vi "DCMotor_WithReduction.vi"(9 "GearBoxReduction":dbl=1.0 format="%13.5p", 11 "in DCMOTOR":T1 {"Jr_KgM2" format="%13.5p"; "L_H" format="%13.5p"; "Kt_NMPerAmp" format="%13.5p"; "KvINV_RadPerSecPerVolt" format="%13.5p"; "R_Ohms" format="%13.5p"; "FreeSpeed_RadPerSec" format="%13.5p"; "FreeCurrent_Amps" format="%13.5p"; "StallCurrent_Amps" format="%13.5p"; "StallTorque_NM" format="%13.5p"; "nominalVoltage_Volts" format="%13.5p"}) -> (3 "out DCMOTOR":T1 {"Jr_KgM2" format="%13.5p"; "L_H" format="%13.5p"; "Kt_NMPerAmp" format="%13.5p"; "KvINV_RadPerSecPerVolt" format="%13.5p"; "R_Ohms" format="%13.5p"; "FreeSpeed_RadPerSec" format="%13.5p"; "FreeCurrent_Amps" format="%13.5p"; "StallCurrent_Amps" format="%13.5p"; "StallTorque_NM" format="%13.5p"; "nominalVoltage_Volts" format="%13.5p"})   [LabVIEW 2019, in "Trajectory_Library.lvlib"]
doc: "Returns a copy of this motor with the given gearbox reduction applied.\n\nInputs: \n - in DCMOTOR -- Cluster containing the motor modeling constants for this set of motors.\n - GearboxReduction -- double -- The gearbox reduction.\n\nOutputs:\n - out DCMOTOR -- Revised cluster containing the motor modeling constants for this set of motors."
uses:
  Trajectory_Library.lvlib
  TypeDef/DCMOTOR.CTL
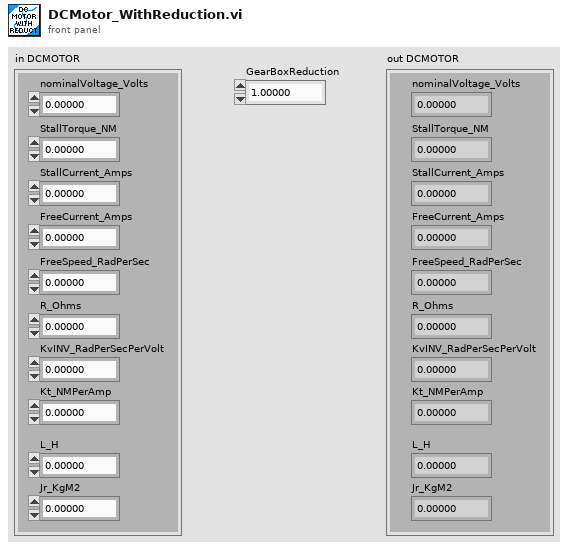
[diagram p1: front panel]
types:
  T1 = typedef "Trajectory_Library.lvlib/DCMOTOR.CTL" = cluster{"nominalVoltage_Volts":dbl, "StallTorque_NM":dbl, "StallCurrent_Amps":dbl, "FreeCurrent_Amps":dbl, "FreeSpeed_RadPerSec":dbl, "R_Ohms":dbl, "KvINV_RadPerSecPerVolt":dbl, "Kt_NMPerAmp":dbl, "L_H":dbl, "Jr_KgM2":dbl}
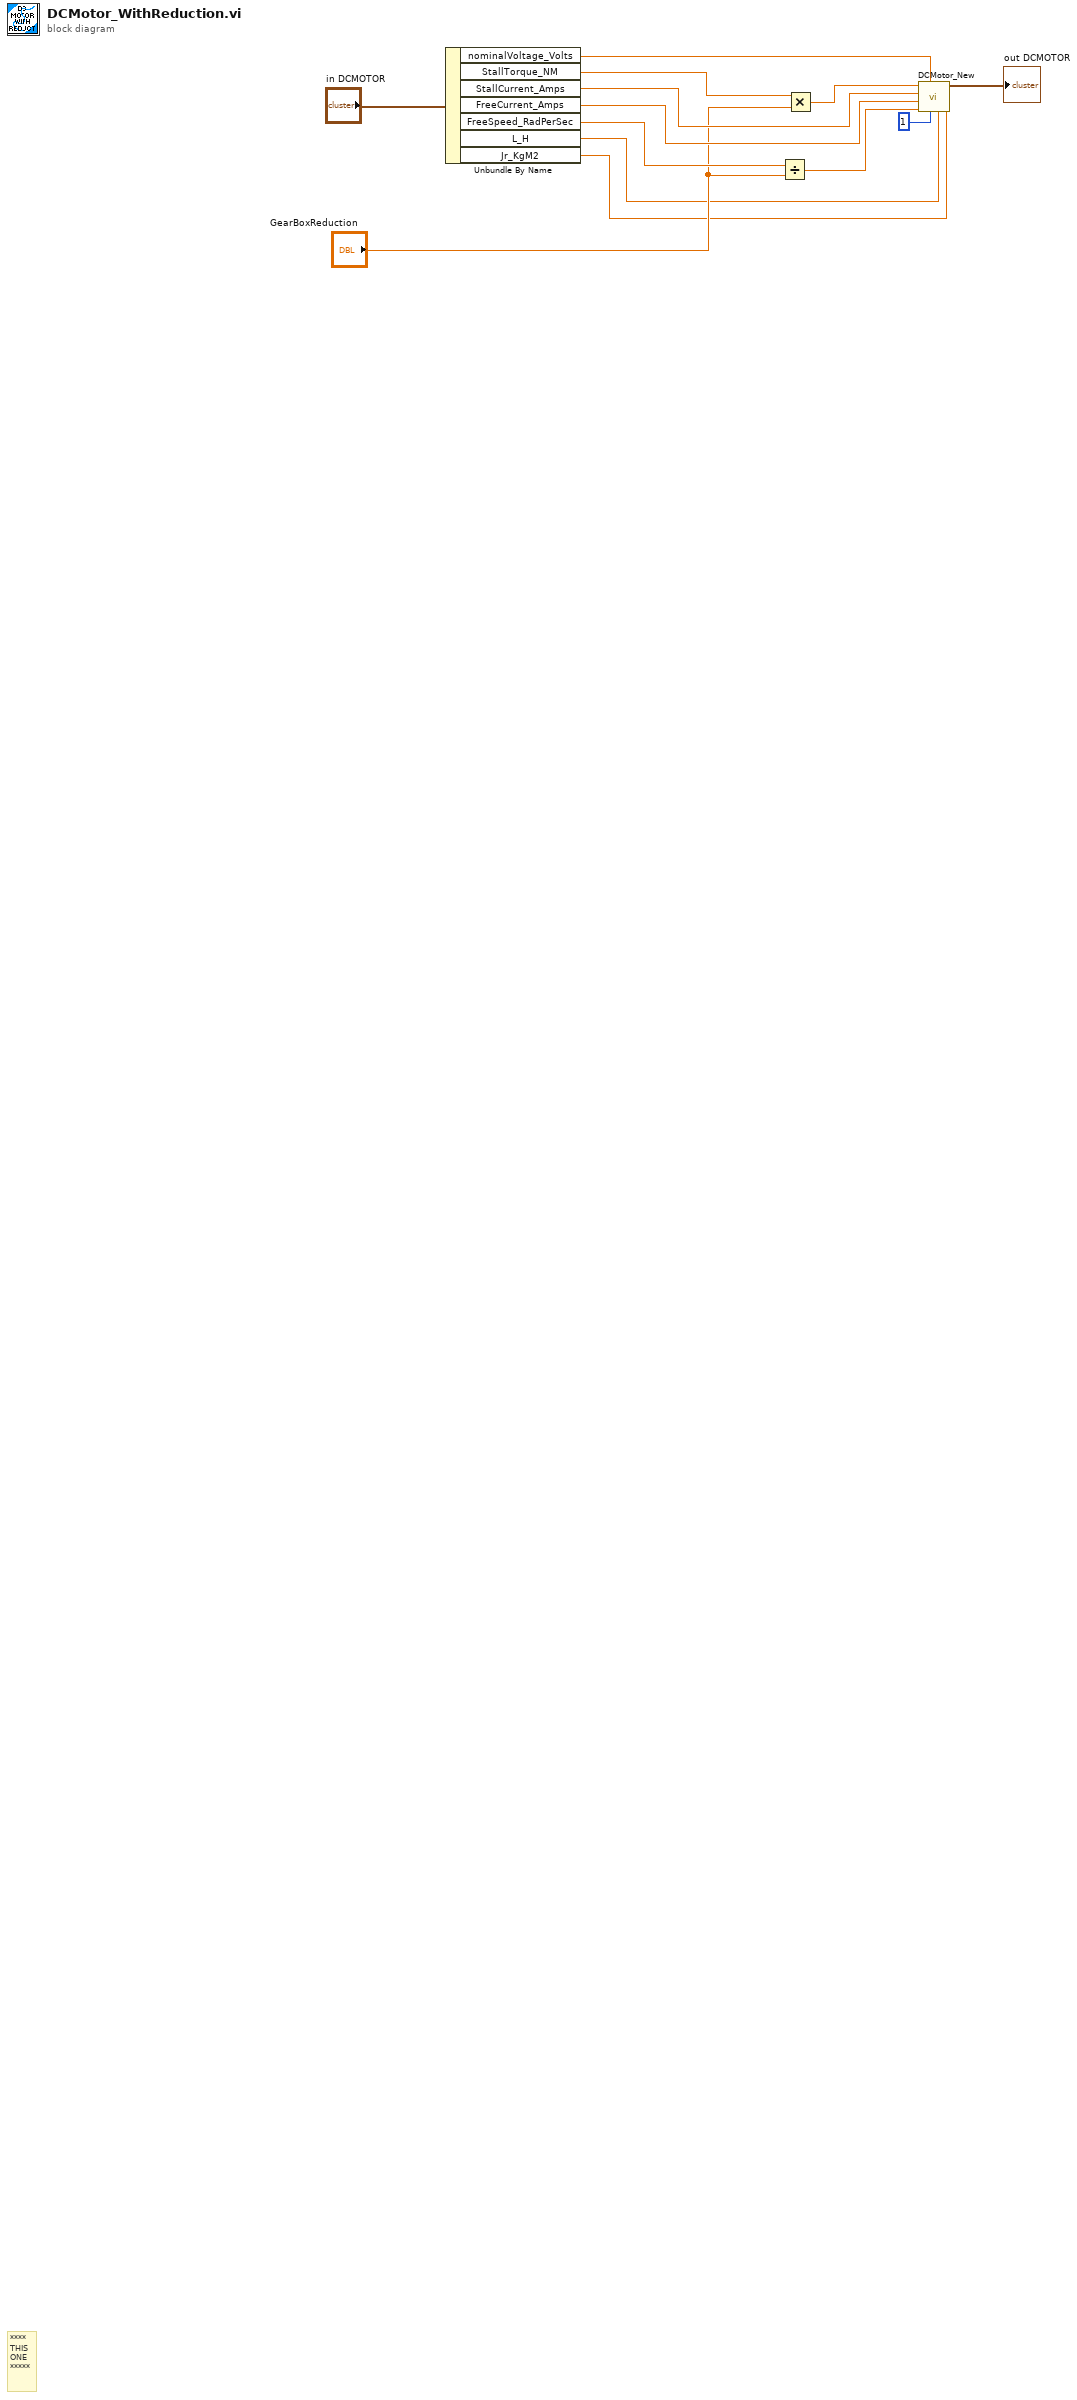
[diagram p0: block diagram]
diagram:
  # "****\nTHIS\nONE\n*****"
  n1 = Unbundle By Name("in DCMOTOR") -> ("nominalVoltage_Volts"=w11:dbl, "StallTorque_NM"=w10:dbl, "StallCurrent_Amps"=w8:dbl, "FreeCurrent_Amps"=w7:dbl, "FreeSpeed_RadPerSec"=w6:dbl, "L_H"=w2:dbl, "Jr_KgM2"=w1:dbl)
  n2 = Divide(x=w6, y="GearBoxReduction") -> (x/y=w4:dbl)
  n3 = Multiply(x=w10, y="GearBoxReduction") -> (x*y=w9:dbl)
  n4 = call "DCMotor_New.vi"("RotorMOI_KgM2"=w1, "Inductance_H"=w2, "Num Motors"=1, "nominalVoltage_Volts"=w11, "FreeSpeed_RadPerSec"=w4, "FreeCurrent_Amps"=w7, "StallCurrent_Amps"=w8, "StallTorque_NM"=w9) -> ("DCMOTOR"=→"out DCMOTOR":T1)  [unwired: 3 in]
